vi "face getslice.vi"(6 "slice type":T1, 7 "reverse? (F)":bool, 8 "error in (no error)":errorcluster, 9 "slice number":u8, 11 "face in":T3) -> (0 "error out":errorcluster, 3 "slice":T2)   [LabVIEW 2011]
uses:
  Typedef/face.ctl
  Typedef/slice.ctl
  Typedef/slice type.ctl
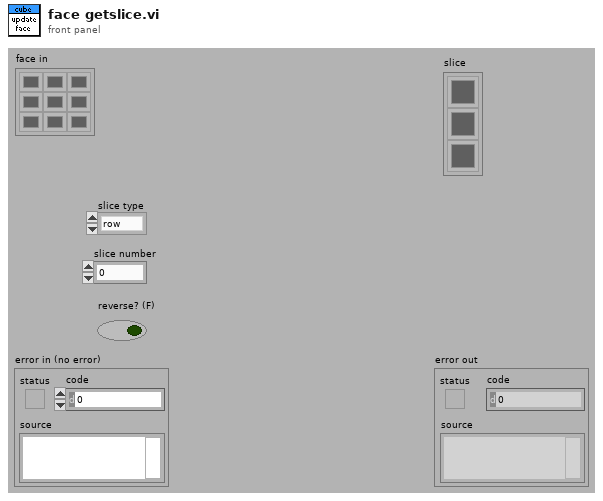
[diagram p1: front panel]
types:
  T1 = typedef "slice type.ctl" = enum16{"row", "col"}
  T2 = typedef "slice.ctl" = u32[]
  T3 = typedef "face.ctl" = u32[][]
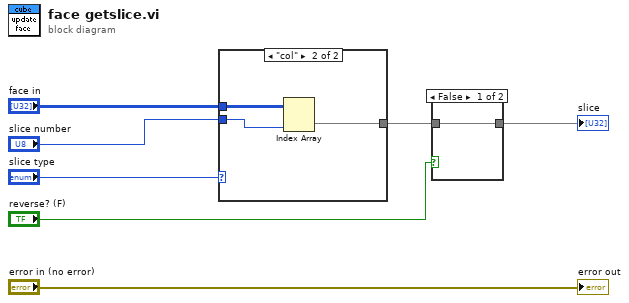
[diagram p0: block diagram]
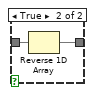
[diagram p2: hidden frame]
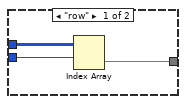
[diagram p3: hidden frame]
diagram:
  n1 = case shown="\"col\"" "slice type" {
    tunnel: "face in" -> [w10 w13]
    tunnel: "slice number" -> [w9 w11]
    tunnel: [w8 w12] -> w2
    frame "row" {
      n2 = Index Array(array=w10, index (row)=w9) -> (element=w8:u32[])  [unwired: 1 in]
    }
    frame "col" {
      n3 = Index Array(array=w13, index (col)=w11) -> (element=w12:u32[])  [unwired: 1 in]
    }
  }
  n4 = case shown="False" "reverse? (F)" {
    tunnel: w2 -> [w14 w16]
    tunnel: [w14 w15] -> w1
    frame False {
    }
    frame True {
      n5 = Reverse 1D Array(array=w16) -> (reversed array=w15:u32[])
    }
  }
  "slice" <- w1
  "error out" <- "error in (no error)"
